vi "Initialize.vi"(8 "error in (no error)":errorcluster caption="错误输入（无错误）") -> (0 "error out":errorcluster caption="错误输出", 2 "function return":i32)   [LabVIEW 2013, in "MvCameraControl.lvlib"]
doc: "MV_LV_API int __stdcall CloseDevice( void* handle);"
uses:
  MvCameraControl.lvlib
  MvCameraControl.dll
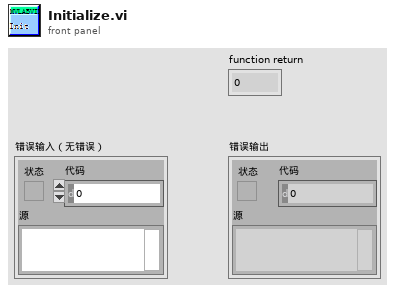
[diagram p1: front panel]
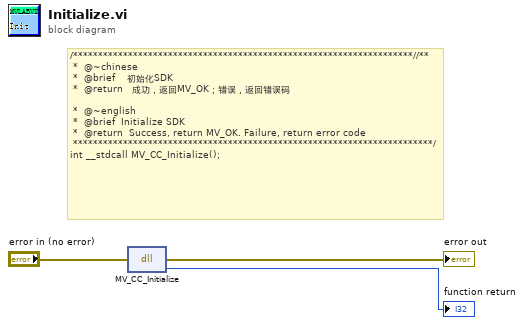
[diagram p0: block diagram]
diagram:
  # "/********************************************************************//**\n *  @~chinese\n *  @brief    初始化SDK\n *  @return   成功，返回MV_OK；错误，返回错误码\n\n *  @~english\n *  @brief  Initialize SDK  \n *  @return  Success, return MV_OK. Failure, return error code   \n ************************************************************************/\nint __stdcall MV_CC_Initialize();"
  n1 = dll-call lib="MvCameraControl.dll" fn="MV_CC_Initialize"(error in="error in (no error)") -> (error out=→"error out":errorcluster, "返回类型"=→"function return":i32)  [unwired: 2 in, 1 out]
